vi "MetodoInit.vi"(7 "Serial Configuration":T1={"Baud Rate"=9600, "Parity"=0, "Stop Bits"=10, "Flow Control"=2} {"Flow Control" items=["None", "XON/XOFF", "RTS/CTS", "XON/XOFF & RTS/CTS", "DTR/DSR", "XON/XOFF & DTR/DSR"]; "Stop Bits" items=["1.0"=10, "1.5"=15, "2.0"=20]; "Parity" items=["None", "Odd", "Even", "Mark", "Space"]; "Baud Rate" items=["300"=300, "600"=600, "1200"=1200, "2400"=2400, "4800"=4800, "9600"=9600, "19200"=19200]}, 8 "error in (no error)":errorcluster, 9 "Reset? (T: Yes)":bool=TRUE, 10 "ID Query? (T: Yes)":bool=TRUE, 11 "TektroniksTDS in":refnum<class "TektroniksTDS.lvclass">) -> (0 "error out":errorcluster, 3 "TektroniksTDS out":refnum<class "TektroniksTDS.lvclass">)   [LabVIEW 2020, in "TektroniksTDS.lvclass"]
uses:
  TektroniksTDS.lvclass
  TektroniksTDS.lvclass/TektroniksTDS.ctl
  <instrlib>/Tektronix TDS 200 1000 2000 Series/Tektronix TDS 200 1000 2000 Series.lvlib
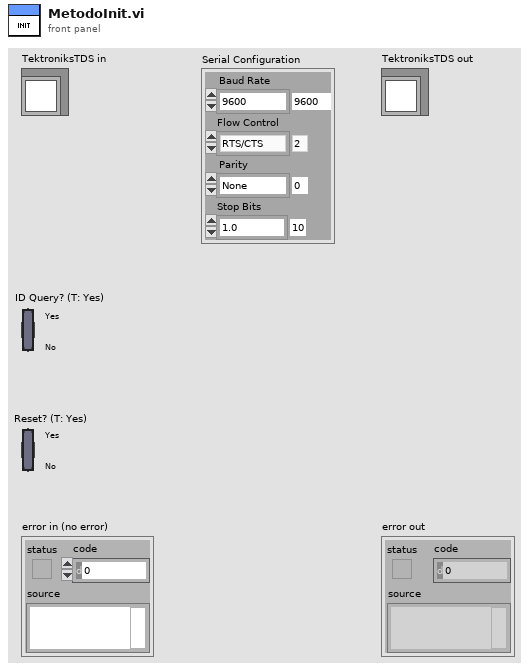
[diagram p1: front panel]
types:
  T1 = cluster{"Baud Rate":u32, "Parity":u16, "Stop Bits":u16, "Flow Control":u16}
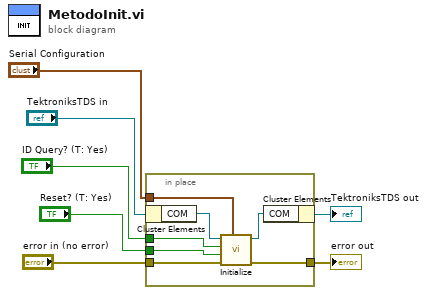
[diagram p0: block diagram]
diagram:
  n1 = in-place {
    in-place-border: "Serial Configuration" -> [w14]
    in-place-border: "ID Query? (T: Yes)" -> [w13]
    in-place-border: "Reset? (T: Yes)" -> [w12]
    in-place-border: "error in (no error)" -> [w11]
    in-place-border: [w10] -> w3
    n2 = in-place-cluster #1("TektroniksTDS in") -> ("COM"=w9:refnum<visa-resource-name>)
    n3 = call <instrlib>:"Initialize.vi"("Serial Configuration"=w14, "error in (no error)"=w11, "Reset? (T: Yes)"=w12, "ID Query? (T: Yes)"=w13, "VISA resource name"=w9) -> ("error out"=w10:errorcluster, "VISA resource name out"=w8:refnum<visa-resource-name>)  [unwired: 5 in]
    n4 = in-place-cluster #1("COM"=w8) -> (→"TektroniksTDS out":refnum<class "TektroniksTDS.lvclass">)
  }
  "error out" <- w3
